vi "Size.vi"(8 "error in (no error)":errorcluster, 11 "Generic Data in":refnum<class "Generic Data.lvclass">) -> (0 "error out":errorcluster, 2 "Size":i32, 3 "Generic Data out":refnum<class "Generic Data.lvclass">)   [LabVIEW 2020, in "Data.lvlib" / "Generic Data.lvclass"]
doc: "Return the size of the generic data element."
uses:
  Generic Data.lvclass
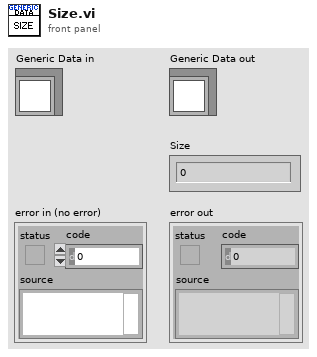
[diagram p1: front panel]
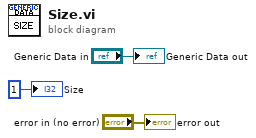
[diagram p0: block diagram]
diagram:
  "error out" <- "error in (no error)"
  "Generic Data out" <- "Generic Data in"
  "Size" <- 1 ("Size")
